vi "_Core(server).vi"(0 "XML config File Path":path=path "D:/work/Project support in lanzhou/OPCUA XML/xml/server config.xml", 7 "error in (no error)":errorcluster, 9 "Op":T1) -> (20 "server endpoint URL":string, 21 "Parse Errors":string, 22 "trusted client certfications":path[](array[path]), 24 "OPC UA server refnum":refnum<k21>, 27 "error out":errorcluster)   [LabVIEW 2014, in "OPCUA Server(UtilityMode)(dev).lvlib"]
uses:
  OPCUA Server(UtilityMode)(dev).lvlib
  _op(server).ctl
  OPCUA XML/OPCUA XML(dev).lvlib
  <vilib>/OPCUA/NI OPC UA Server.lvlib
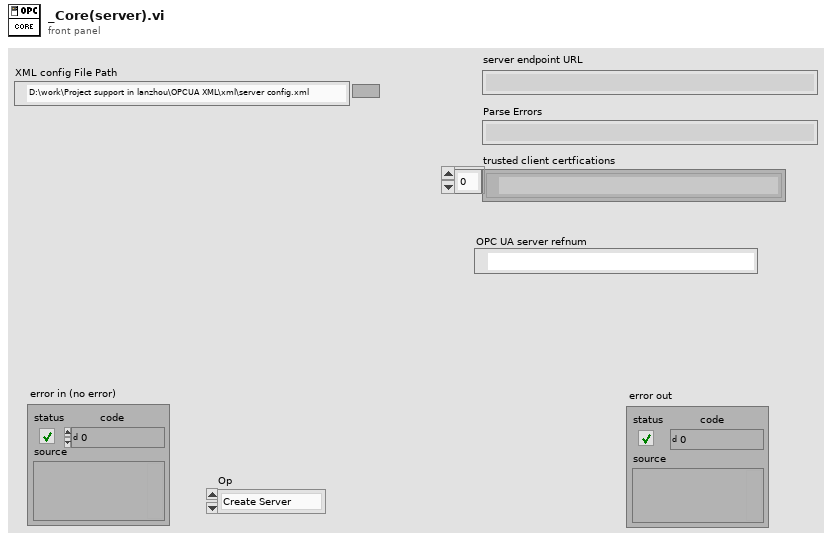
[diagram p1: front panel]
types:
  T1 = typedef "OPCUA Server(UtilityMode)(dev).lvlib/_op(server).ctl" = enum16{"Create Server", "Start Server", "Get Server Refnum", "Stop Server", "Close Server"}
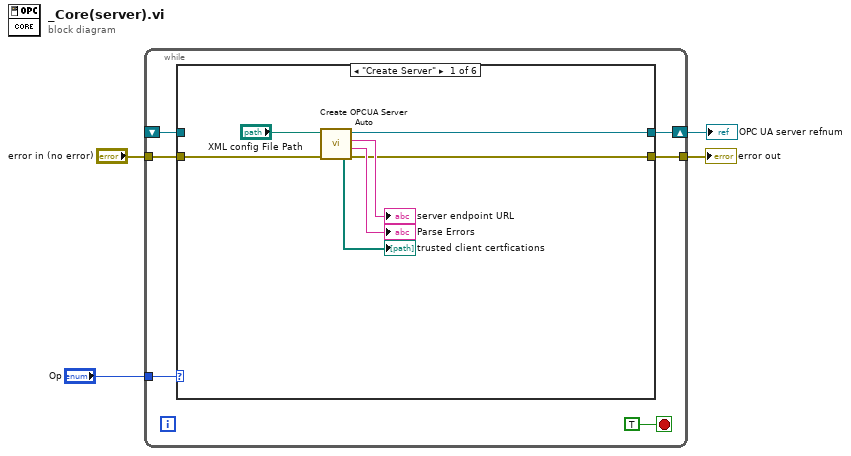
[diagram p0: block diagram]
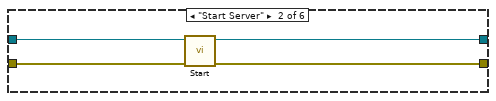
[diagram p2: hidden frame]
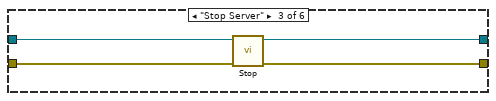
[diagram p3: hidden frame]
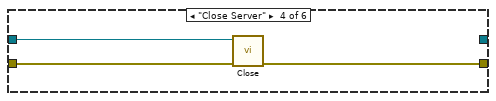
[diagram p4: hidden frame]
diagram:
  n1 = while {
    tunnel: "Op" -> [w9]
    shift-right: [w7] -> w1
    shift-left: _ -> [w8]
    tunnel: [w6] -> w2
    tunnel: "error in (no error)" -> [w5]
    stop <- TRUE stop-if-true
    n2 = case shown="\"Create Server\"" w9 {
      tunnel: w8 -> [_ w21 w23 w28 w30 w32]
      tunnel: [w14 w18 w25 _ w30 w32] -> w7
      tunnel: [w13 w19 w24 w26 w29 w31] -> w6
      tunnel: w5 -> [w12 w20 w22 w27 w29 w31]
      frame "Create Server" {
        n3 = call "Create OPCUA Server Auto.vi"("Error In"=w12, "XML config File Path"="XML config File Path") -> ("Error Out"=w13:errorcluster, "Parse Errors"=→"Parse Errors":string, "server endpoint URL"=→"server endpoint URL":string, "OPC UA server refnum out"=w14:refnum<k21>, "trusted client certfications"=→"trusted client certfications":path[])  [unwired: 5 in]
      }
      frame "Start Server" {
        n4 = call <vilib>:"Start.vi"("error in (no error)"=w20, "OPC UA server refnum in"=w21) -> ("error out"=w19:errorcluster, "OPC UA server refnum out"=w18:refnum<k21>)  [unwired: 8 in]
      }
      frame "Stop Server" {
        n5 = call <vilib>:"Stop.vi"("error in (no error)"=w22, "OPC UA server refnum in"=w23) -> ("error out"=w24:errorcluster, "OPC UA server refnum out"=w25:refnum<k21>)  [unwired: 8 in]
      }
      frame "Close Server" {
        n6 = call <vilib>:"Close.vi"("error in (no error)"=w27, "OPC UA server refnum in"=w28) -> ("error out"=w26:errorcluster)  [unwired: 9 in]
      }
      frame Default {
      }
      frame "Get Server Refnum" {
      }
    }
  }
  "error out" <- w2
  "OPC UA server refnum" <- w1
